vi "RunSieve.vi"(8 "error in (no error)":errorcluster, 11 "Prime_Sieve in":refnum<class "Prime_Sieve.lvclass">) -> (0 "error out":errorcluster, 3 "Prime_Sieve out":refnum<class "Prime_Sieve.lvclass">)   [LabVIEW 2020, in "Prime_Sieve.lvclass"]
uses:
  Prime_Sieve.lvclass
  Prime_Sieve.lvclass/Prime_Sieve.ctl
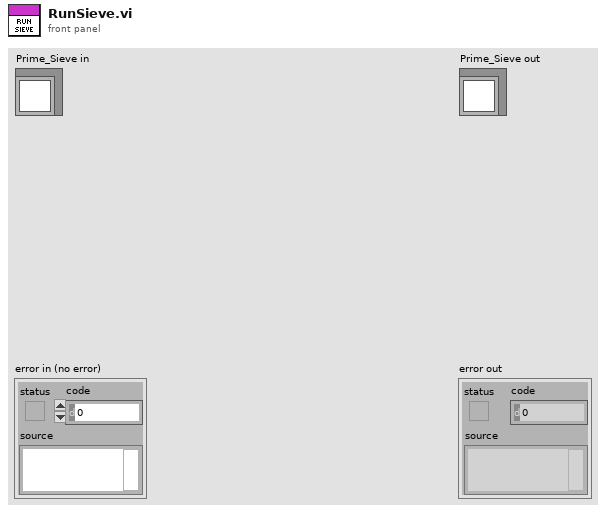
[diagram p1: front panel]
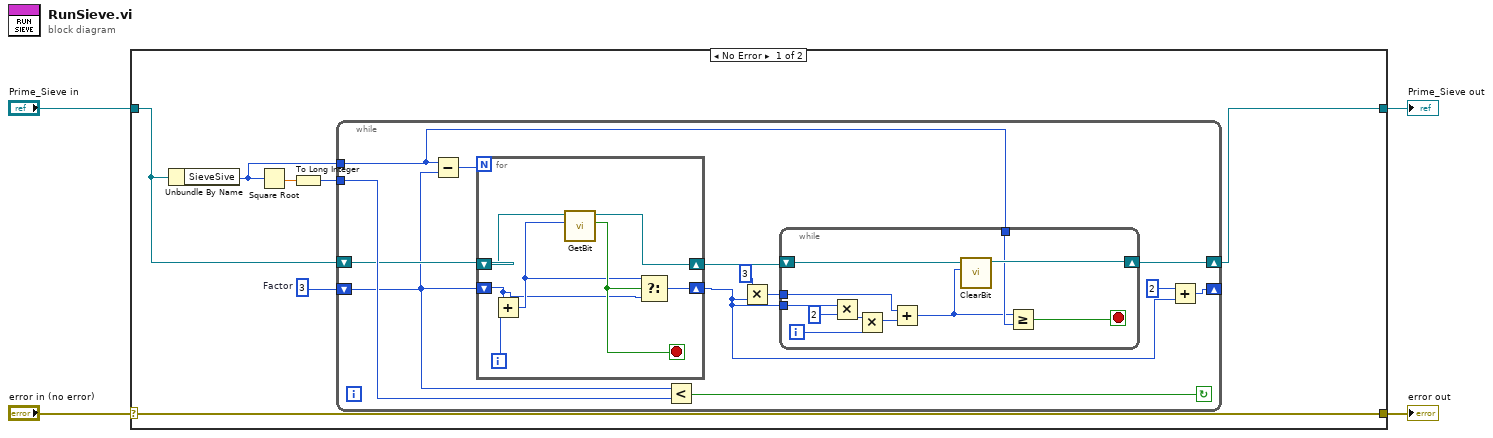
[diagram p0: block diagram]
diagram:
  n1 = case shown="No Error" "error in (no error)" {
    selector: "error in (no error)" -> [w11 w44]
    tunnel: [w11 w44] -> w3
    tunnel: [w6 w43] -> w1
    tunnel: "Prime_Sieve in" -> [w5 w43]
    frame No Error {
      w9 = 3  # Factor
      n2 = Unbundle By Name(w5) -> ("SieveSive"=w8:i64)
      n3 = Square Root(x=w8) -> (sqrt(x)=w10:dbl)
      n4 = To Long Integer(number=w10) -> (32bit integer=w7:i32)
      n5 = while {
        tunnel: w8 -> [w16]
        shift-right: [w19] -> _
        shift-left: w9 -> [w15]
        tunnel: w7 -> [w23]
        shift-right: [w18] -> w6
        shift-left: w5 -> [w22]
        stop <- w24 continue-if-true
        n6 = Subtract(x=w16, y=w15) -> (x-y=w17:i64)
        n7 = for {
          N: w17 -> [_]
          shift-right: [w30] -> w21
          shift-left: w22 -> [w31]
          shift-right: [w29] -> w13
          shift-left: w15 -> [w25]
          i -> [w27]
          stop <- w28 stop-if-true
          n8 = Add(x=w25, y=w27) -> (x+y=w26:i32)
          n9 = call "GetBit.vi"("Index"=w26, "Prime_Sieve in"=w31) -> ("Boolean"=w28:bool, "Prime_Sieve out"=w30:refnum<class "Prime_Sieve.lvclass">)  [unwired: 7 in, 1 out]
          n10 = Select(t=w26, s=w28, f=w25) -> (s? t:f=w29:i32)
        }
        n11 = Less?(x=w15, y=w23) -> (x < y?=w24:bool)
        n12 = Multiply(x=3 ("y"), y=w13) -> (x*y=w14:i32)
        n13 = while {
          shift-right: [w41] -> w18
          shift-left: w21 -> [w42]
          tunnel: w16 -> [w40]
          tunnel: w14 -> [w33]
          tunnel: w13 -> [w37]
          i -> [w35]
          stop <- w38 stop-if-true
          n14 = Multiply(x=w37, y=2) -> (x*y=w36:i32)
          n15 = Multiply(x=w36, y=w35) -> (x*y=w34:i32)
          n16 = Add(x=w33, y=w34) -> (x+y=w32:i32)
          n17 = call "ClearBit.vi"("Index"=w32, "Prime_Sieve in"=w42) -> ("Prime_Sieve out"=w41:refnum<class "Prime_Sieve.lvclass">)  [unwired: 8 in, 1 out]
          n18 = Greater Or Equal?(x=w32, y=w40) -> (x >= y?=w38:bool)
        }
        n19 = Add(x=2, y=w13) -> (x+y=w19:i32)
      }
    }
    frame Error {
    }
  }
  "error out" <- w3
  "Prime_Sieve out" <- w1
